vi "dfd_ZPK to TF.vi"(9 "gain":dbl=1.0, 10 "poles":cdb[](array[numeric]), 11 "zeros":cdb[](array[numeric])) -> (2 "denominator":dbl[](array[numeric]) format="%.2f", 3 "numerator":dbl[](array[numeric]) format="%.2f")   [LabVIEW 2017, in "NI_DigFilterLicensed.lvlib"]
uses:
  <vilib>/addons/Digital Filter Design/NI_DigFilterLicensed.lvlib
  <vilib>/Analysis/polynomials.llb/Create Polynomial From Roots (CDB).vi
  <vilib>/Analysis/NI_AALPro.lvlib
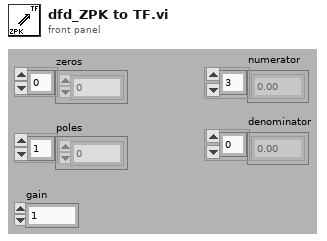
[diagram p1: front panel]
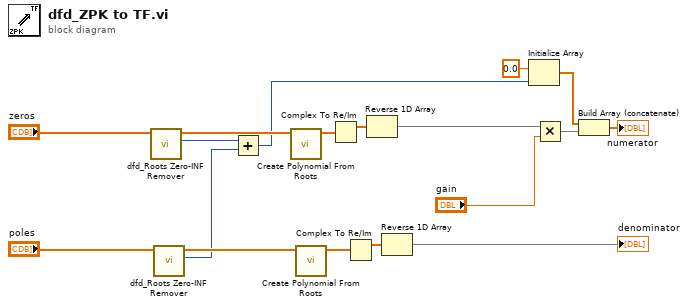
[diagram p0: block diagram]
diagram:
  n1 = call <vilib>:"dfd_Roots Zero-INF Remover.vi"("roots"="zeros") -> ("# zero root"=w3:i32, "new roots"=w7:cdb[])  [unwired: 9 out]
  n2 = call <vilib>:"dfd_Roots Zero-INF Remover.vi"("roots"="poles") -> ("# zero root"=w2:i32, "new roots"=w8:cdb[])  [unwired: 9 out]
  n3 = Add(x=w3, y=w2) -> (x+y=w4:i32)
  n4 = call-poly <vilib>:"Create Polynomial From Roots.vi"("Roots"=w7) -> ("P(x)"=w17:cdb[])  [unwired: 10 out]
  n5 = call-poly <vilib>:"Create Polynomial From Roots.vi"("Roots"=w8) -> ("P(x)"=w12:cdb[])  [unwired: 10 out]
  n6 = Complex To Re/Im(x + iy=w17) -> (x=w16:dbl[])  [unwired: 1 out]
  n7 = Complex To Re/Im(x + iy=w12) -> (x=w13:dbl[])  [unwired: 1 out]
  n8 = Reverse 1D Array(array=w16) -> (reversed array=w6:dbl[])
  n9 = Reverse 1D Array(array=w13) -> (reversed array=→"denominator":dbl[])
  n10 = Initialize Array(0.0 ("element"), w4) -> (w9:dbl[])
  n11 = Multiply(x=w6, y="gain") -> (x*y=w14:dbl[])
  n12 = Build Array (concatenate)(w9, w14) -> (→"numerator":dbl[])
